vi "Keysight66332A.vi"(4 "error in":T13, 7 "Command":T14) -> (0 "error out":T13, 3 "Response":T11)   [LabVIEW 2018]
uses:
  MOKO_LabViewLibrary/MokoLowLevel/MokoLowLovelControl/MLLC_Command.ctl
  MOKO_LabViewLibrary/MokoLowLevel/MokoLowLovelControl/MLLC_Error.ctl
  MOKO_LabViewLibrary/MokoLowLevel/MokoLowLovelControl/MLLC_Mode.ctl
  MOKO_LabViewLibrary/MokoLowLevel/MokoLowLovelControl/MLLC_Response.ctl
  MOKO_LabViewLibrary/MokoLowLevel/MokoLowLovelControl/MLLC_DriverName.ctl
  MOKO_LabViewLibrary/MokoLowLevel/MokoLowLovelControl/MLLC_Request.ctl
  MOKO_LabViewLibrary/MokoLowLevel/MokoLowLovelControl/MLLC_ErrorCode.ctl
  MOKO_LabViewLibrary/MokoLowLevel/MokoLowLovelControl/MLLC_ResponseInit.ctl
  MOKO_LabViewLibrary/MokoLowLevel/MokoLowLovelControl/MLLC_ConnectCluster.ctl
  MOKO_LabViewLibrary/MokoLowLevel/MokoLowLovelControl/MLLC_InterfaceType.ctl
  MOKO_LabViewLibrary/MokoLowLevel/MokoLowLovelControl/MLLC_OpenedSession.ctl
  MOKO_LabViewLibrary/MokoLowLevel/MokoLowLovelControl/MLLC_InterfaceSettings.ctl
  MOKO_LabViewLibrary/MokoLowLevel/MokoLowLovelControl/MLLC_InterfaceKind.ctl
panel:
  in  "Settings":T6={"Saved Data"=variant, "Data"={"Connect"={"InterfaceType"=enum."VISA", "OpenedSession"="", "InterfaceSettings"={"Interface"=enum."GPIB", "EOS 4 read"=enum."LF (\\n)", "EOS 4 write"=enum."LF (\\n)", "TMO, ms"=5000, "Sett"=variant(cluster{"Baud Rate":u32, "Data Bits":u16, "Parity":u16, "Stop Bits":u16, "Flow Control":u16, "Eho":bool} {"Baud Rate"=75, "Data Bits"=0, "Parity"=0, "Stop Bits"=0, "Flow Control"=0, "Eho"=FALSE})}}, "VDC Range"=FALSE}}
  in  "Response":T7="663"
  in  "Error Code":T8=5475
  in  "Request":T9="*idn?"
  in  "Driver Name":T10="Keysight6632B"
  in  "Mode":T12=enum."Check"
  # ":VOLT:RANG LOW"
  # ":VOLT 5.000"
  # "SCPI = *RST"
  # "Keysight66332A"
  # "SCPI =OUTPut OFF"
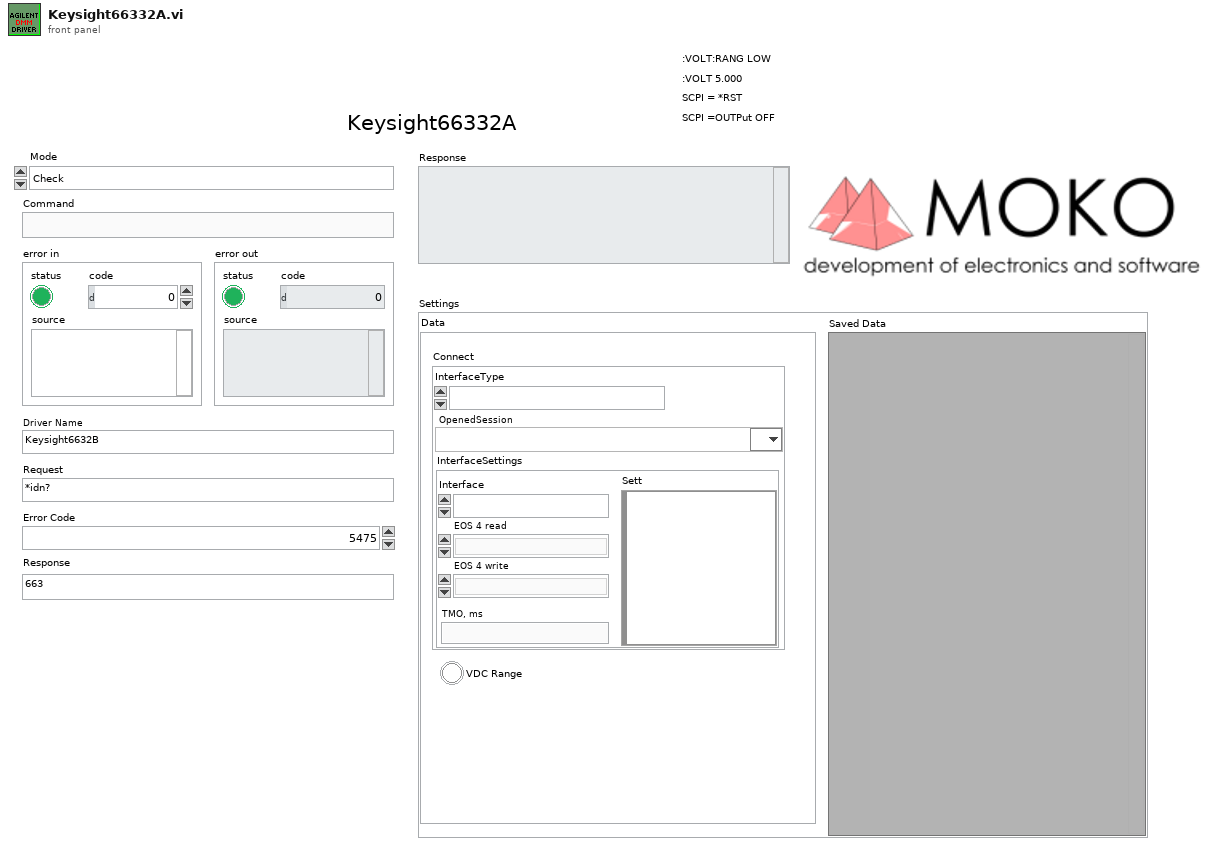
[diagram p1: front panel]
types:
  T1 = typedef "MLLC_ConnectCluster.ctl" = cluster{"InterfaceType":T2, "OpenedSession":T3, "InterfaceSettings":T4}
  T2 = typedef "MLLC_InterfaceType.ctl" = enum16{"VISA", "Prologix USB-GPIB"}
  T3 = typedef "MLLC_OpenedSession.ctl" = refnum<visa-resource-name>
  T4 = typedef "MLLC_InterfaceSettings.ctl" = cluster{"Interface":T5, "EOS 4 read":enum16{"Default (=EOS 4 write)", "CR (\\r)", "LF (\\n)", "None"}, "EOS 4 write":enum16{"CR+LF (\\r\\n)", "CR (\\r)", "LF (\\n)", "None"}, "TMO, ms":i32, "Sett":variant}
  T5 = typedef "MLLC_InterfaceKind.ctl" = enum16{"RS232", "GPIB", "USB", "Ethernet", "another"}
  T6 = cluster{"Saved Data":variant, "Data":cluster{"Connect":T1, "VDC Range":bool}}
  T7 = typedef "MLLC_ResponseInit.ctl" = string
  T8 = typedef "MLLC_ErrorCode.ctl" = u32
  T9 = typedef "MLLC_Request.ctl" = string
  T10 = typedef "MLLC_DriverName.ctl" = string
  T11 = typedef "MLLC_Response.ctl" = string
  T12 = typedef "MLLC_Mode.ctl" = enum16{"get", "set", "close", "Init", "Check"}
  T13 = typedef "MLLC_Error.ctl" = errorcluster
  T14 = typedef "MLLC_Command.ctl" = string
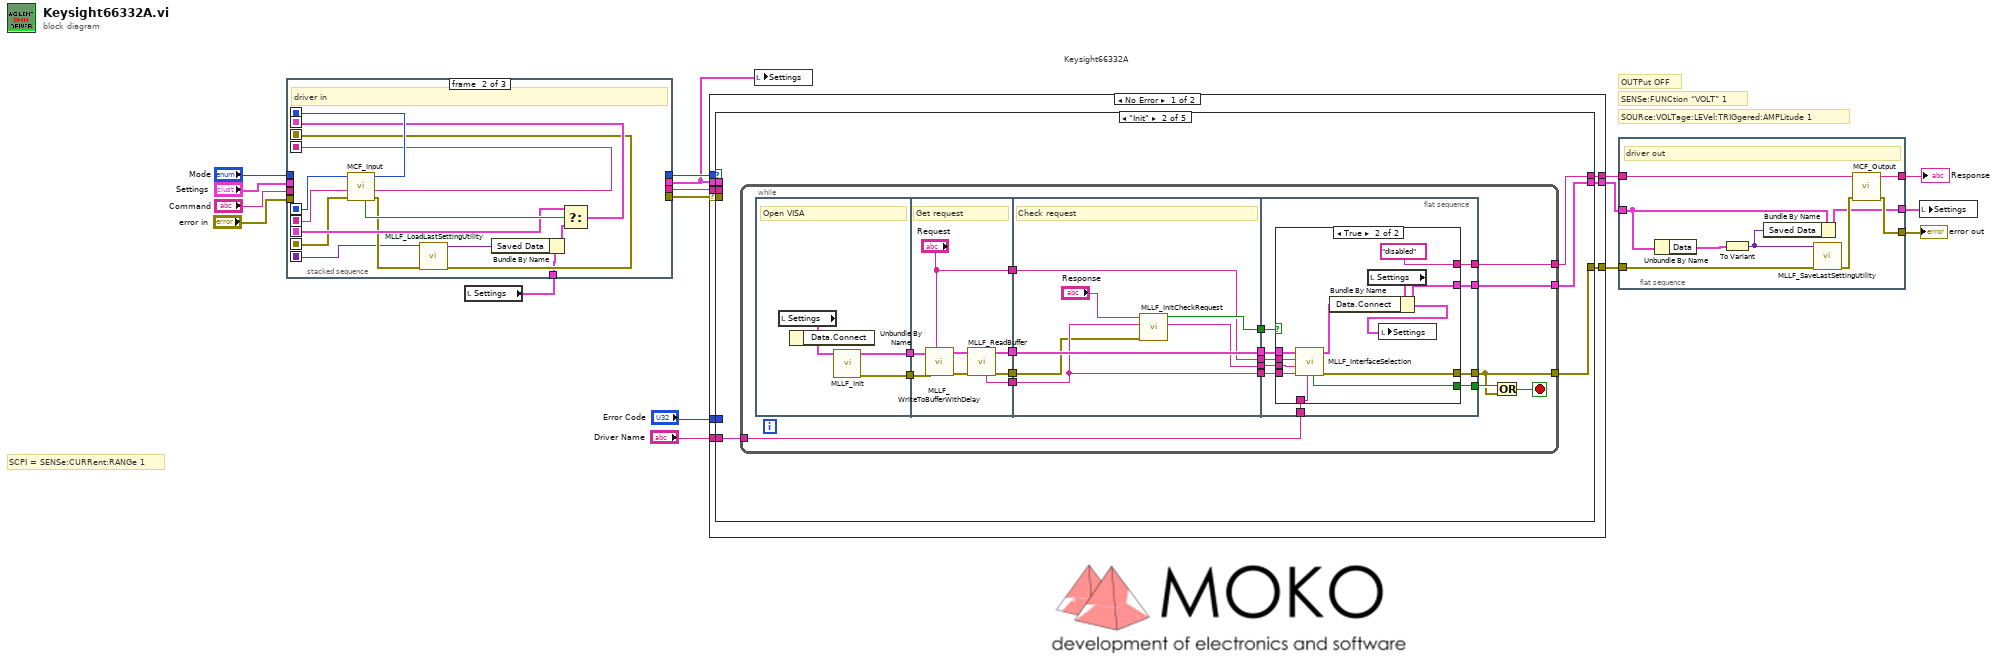
[diagram p0: block diagram]
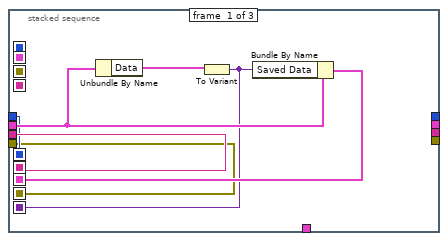
[diagram p2: hidden frame]
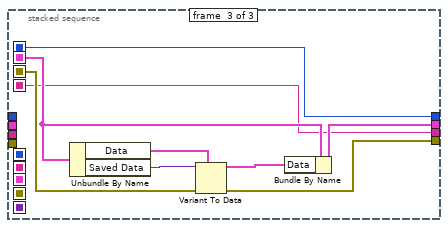
[diagram p3: hidden frame]
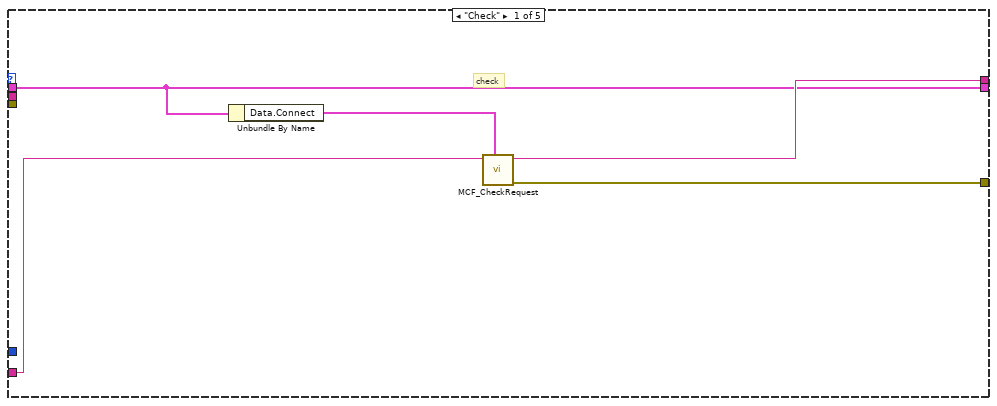
[diagram p4: hidden frame]
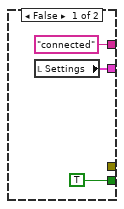
[diagram p5: hidden frame]
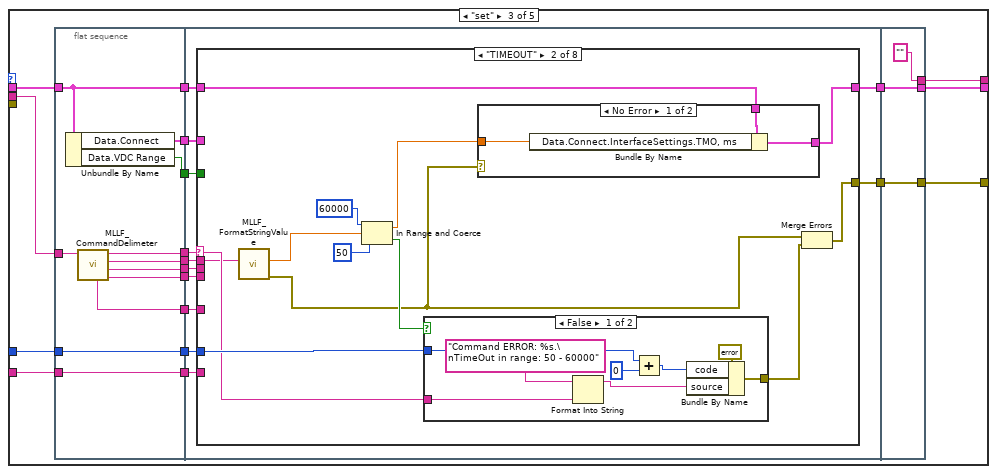
[diagram p6: hidden frame]
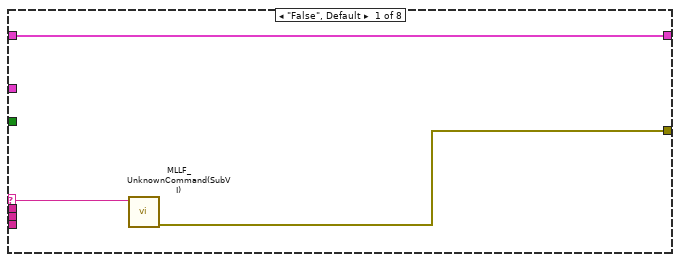
[diagram p7: hidden frame]
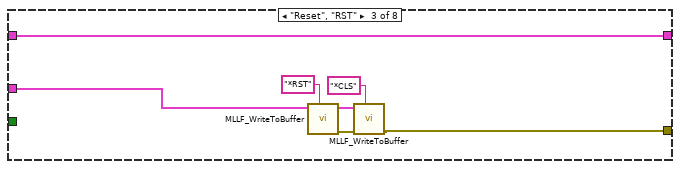
[diagram p10: hidden frame]
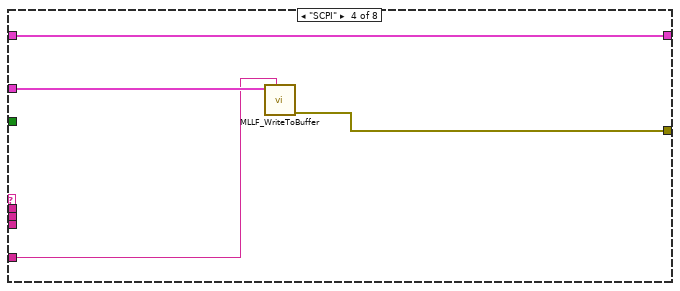
[diagram p11: hidden frame]
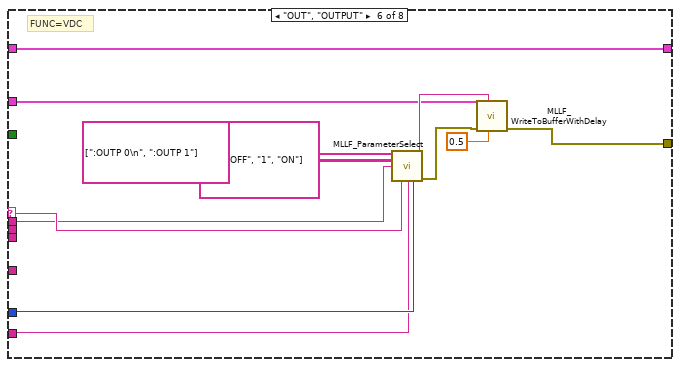
[diagram p13: hidden frame]
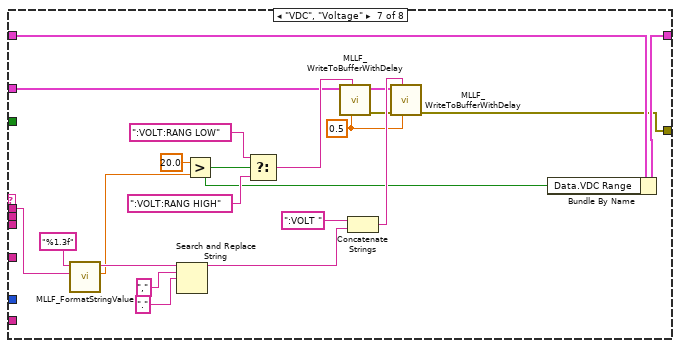
[diagram p14: hidden frame]
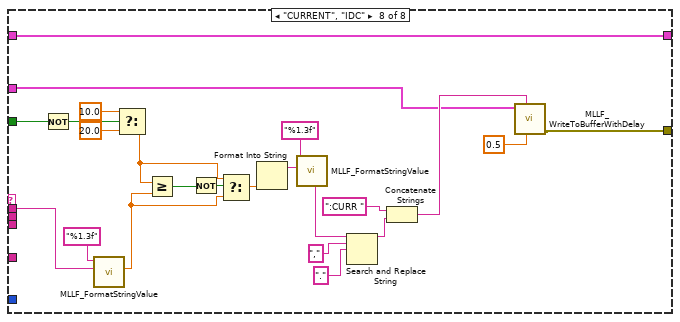
[diagram p15: hidden frame]
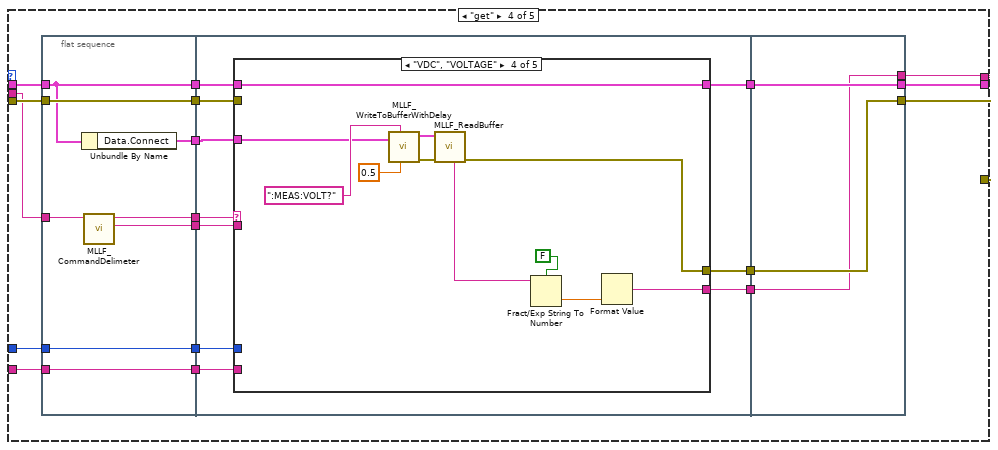
[diagram p16: hidden frame]
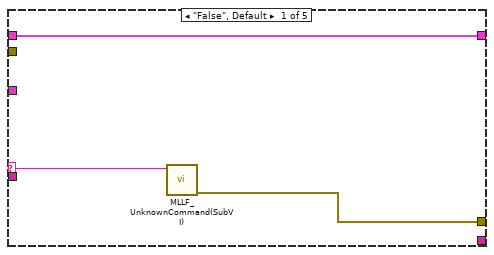
[diagram p17: hidden frame]
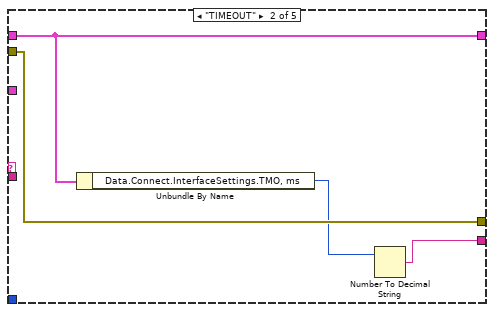
[diagram p18: hidden frame]
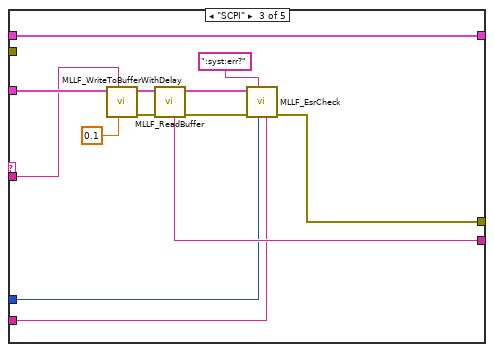
[diagram p19: hidden frame]
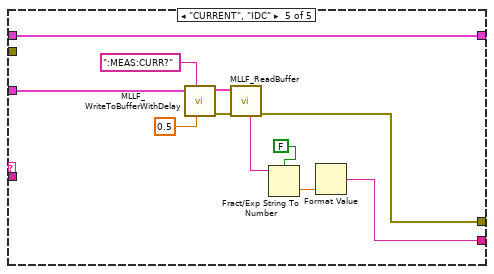
[diagram p20: hidden frame]
diagram:
  # "OUTPut OFF"
  # "SOURce:VOLTage:LEVel:TRIGgered:AMPLitude 1"
  # "SENSe:FUNCtion “VOLT” 1"
  # "SCPI = SENSe:CURRent:RANGe 1"
  # "Keysight66332A"
  n1 = local read "Settings"() -> (w8:T6)
  n2 = stacked-sequence {
    seq-local: [w20 _ _] -> [_ w36 _]
    seq-local: [w19 _ _] -> [_ w37 _]
    seq-local: [w22 _ _] -> [_ w32 _]
    seq-local: [w18 _ _] -> [_ w31 _]
    seq-local: [w21 _ _] -> [_ w27 _]
    seq-local: [_ w28 _] -> [_ _ w44]
    seq-local: [_ w38 _] -> [_ _ w41]
    seq-local: [_ w35 _] -> [_ _ w40]
    seq-local: [_ w34 _] -> [_ _ w45]
    tunnel: "Command" -> [w20 _ _]
    tunnel: "Mode" -> [w19 _ _]
    tunnel: "error in" -> [w18 _ _]
    tunnel: "Settings" -> [w23 _ _]
    tunnel: w8 -> [_ w26 _]
    tunnel: [_ _ w40] -> w10
    tunnel: [_ _ w43] -> w1
    tunnel: [_ _ w42] -> w9
    tunnel: [_ _ w41] -> w11
    frame #0 {
      n3 = Unbundle By Name(w23) -> ("Data"=w24:cluster{"Connect":T1, "VDC Range":bool})
      n4 = To Variant(anything=w24) -> (Variant=w21:variant)
      n5 = Bundle By Name(cluster=w23, "Saved Data"=w21) -> (w22:T6)
    }
    frame #1 {
      # "driver in"
      n6 = call "MCF_Input.vi"("Error In"=w31, "Command in"=w36, "Mode in"=w37) -> ("Error Out"=w30:errorcluster, "Command out"=w35:string, "Mode out"=w38:T12, "Boolean"=w33:bool)  [unwired: 5 in]
      n7 = call "MLLF_LoadLastSettingUtility.vi"("Error In"=w30, "Save data in"=w27) -> ("Error Out"=w28:errorcluster, "Save data out"=w25:variant)  [unwired: 8 in]
      n8 = Bundle By Name(cluster=w26, "Saved Data"=w25) -> (w29:T6)
      n9 = Select(t=w32, s=w33, f=w29) -> (s? t:f=w34:T6)
    }
    frame #2 {
      n10 = Unbundle By Name(w45) -> ("Data"=w46:cluster{"Connect":T1, "VDC Range":bool}, "Saved Data"=w39:variant)
      n11 = Variant To Data(error in=w44, type=w46, Variant=w39) -> (data=w47:cluster{"Connect":T1, "VDC Range":bool}, error out=w42:errorcluster)
      n12 = Bundle By Name(cluster=w45, "Data"=w47) -> (w43:T6)
    }
  }
  n13 = case shown="No Error" w9 {
    selector: w9 -> [w53 w354]
    tunnel: [w54 w354] -> w5
    tunnel: w11 -> [w56 _]
    tunnel: [w55 "An error occurred in the driver input module." ("String")] -> w7
    tunnel: w10 -> [w48 _]
    tunnel: w1 -> [w49 w353]
    tunnel: "Error Code" -> [w52 _]
    tunnel: "Driver Name" -> [w51 _]
    tunnel: [w50 w353] -> w6
    frame No Error {
      n14 = case shown="\"Init\"" w56 {
        tunnel: [w60 w65 w138 w267 "" ("String")] -> w55
        tunnel: [w61 w63 w141 w268 w350] -> w54
        tunnel: w53 -> [_ _ _ w281 _]
        tunnel: w52 -> [_ _ w144 w283 _]
        tunnel: w51 -> [w59 w62 w142 w282 _]
        tunnel: [w57 w64 w143 w284 w349] -> w50
        tunnel: w49 -> [w57 _ w129 w273 w349]
        tunnel: w48 -> [_ _ w128 w272 _]
        frame "Check" {
          # "check"
          n15 = Unbundle By Name(w57) -> ("Data.Connect"=w58:T1)
          n16 = call "MCF_CheckRequest.vi"("Permanent data.Connect"=w58, "Driver Name"=w59) -> ("Error Out"=w61:errorcluster, "Output String"=w60:string)  [unwired: 8 in]
        }
        frame "Init" {
          n17 = while {
            tunnel: [w71] -> w63
            tunnel: [w70] -> w65
            tunnel: [w69] -> w64
            tunnel: w62 -> [w73]
            stop <- w82 stop-if-true
            n18 = flat-sequence {
              tunnel: [w86] -> w81
              tunnel: [w85] -> w80
              tunnel: w81 -> [w92]
              tunnel: w80 -> [w91]
              tunnel: [w90] -> w79
              tunnel: [w89] -> w78
              tunnel: [w88] -> w77
              tunnel: ["Request"] -> w67
              tunnel: w79 -> [w98]
              tunnel: w78 -> [w101]
              tunnel: w77 -> [w100]
              tunnel: [w101] -> w76
              tunnel: [w100] -> w75
              tunnel: [w97] -> w74
              tunnel: [w96] -> w68
              tunnel: w67 -> [w95]
              tunnel: [w95] -> w66
              tunnel: w76 -> [w110]
              tunnel: w75 -> [w109]
              tunnel: w74 -> [w111]
              tunnel: w73 -> [w108]
              tunnel: [w107] -> w72
              tunnel: [w106] -> w71
              tunnel: [w105] -> w70
              tunnel: [w104] -> w69
              tunnel: w68 -> [w103]
              tunnel: w66 -> [w102]
              frame #0 {
                # "Open VISA"
                n19 = local read "Settings"() -> (w84:T6)
                n20 = Unbundle By Name(w84) -> ("Data.Connect"=w83:T1)
                n21 = call "MLLF_Init.vi"("DriverConnect in"=w83) -> ("Error Out"=w86:errorcluster, "DriverConnect out"=w85:T1)  [unwired: 7 in]
              }
              frame #1 {
                # "Get request"
                n22 = call "MLLF_WriteToBufferWithDelay.vi"("Command"="Request", "Error In"=w92, "DriverConnect in"=w91) -> ("Error Out"=w93:errorcluster, "DriverConnect out"=w94:T1)  [unwired: 7 in]
                n23 = call "MLLF_ReadBuffer.vi"("Error In"=w93, "DriverConnect in"=w94) -> ("Error Out"=w90:errorcluster, "DriverConnect out"=w89:T1, "String"=w88:string)  [unwired: 6 in]
              }
              frame #2 {
                # "Check request"
                n24 = call "MLLF_InitCheckRequest.vi"("error in (no error)"=w98, "Answer"=w100, "Response Init"="Response") -> ("ResponseInit out"=w96:string, "Design"=w97:bool)  [unwired: 5 in, 2 out]
              }
              frame #3 {
                n25 = case shown="True" w111 {
                  tunnel: w110 -> [_ w124]
                  tunnel: [TRUE w119] -> w107
                  tunnel: [_ w122] -> w106
                  tunnel: ["connected" "disabled"] -> w105
                  tunnel: [w112 w120] -> w104
                  tunnel: w109 -> [_ w117]
                  tunnel: w108 -> [_ w118]
                  tunnel: w103 -> [_ w116]
                  tunnel: w102 -> [_ w115]
                  frame False {
                    n26 = local read "Settings"() -> (w112:T6)
                  }
                  frame True {
                    n27 = call "MLLF_InterfaceSelection.vi"("Driver Name"=w118, "Answer:"=w117, "Response"=w116, "Request"=w115, "DriverConnect in"=w124) -> ("error out"=w122:T13, "DriverConnect out"=w123:T1, "stop init?"=w119:bool)  [unwired: 2 in, 2 out]
                    n28 = local read "Settings"() -> (w125:T6)
                    n29 = Bundle By Name(cluster=w125, "Data.Connect"=w123) -> (w120:T6)
                    n30 = local write "Settings"(w120) -> ()
                  }
                }
              }
            }
            n31 = Or(x=w72, y=w71) -> (x .or. y?=w82:bool)
          }
        }
        frame "set" {
          n32 = flat-sequence {
            tunnel: w142 -> [w154]
            tunnel: w129 -> [w147]
            tunnel: w144 -> [w155]
            tunnel: [w155] -> w137
            tunnel: [w147] -> w136
            tunnel: [w154] -> w135
            tunnel: [w153] -> w134
            tunnel: [w148] -> w133
            tunnel: [w149] -> w132
            tunnel: [w150] -> w131
            tunnel: [w151] -> w130
            tunnel: w128 -> [w152]
            tunnel: [w146] -> w127
            tunnel: [w145] -> w126
            tunnel: [w165] -> w140
            tunnel: [w160] -> w139
            tunnel: w137 -> [w167]
            tunnel: w136 -> [w166]
            tunnel: w135 -> [w164]
            tunnel: w134 -> [w163]
            tunnel: w133 -> [w162]
            tunnel: w132 -> [w161]
            tunnel: w131 -> [w159]
            tunnel: w130 -> [w158]
            tunnel: w127 -> [w157]
            tunnel: w126 -> [w156]
            tunnel: [w265] -> w141
            tunnel: [w266] -> w143
            tunnel: w140 -> [w266]
            tunnel: w139 -> [w265]
            tunnel: ["" ("String")] -> w138
            frame #0 {
              n33 = Unbundle By Name(w147) -> ("Data.Connect"=w153:T1, "Data.VDC Range"=w145:bool)
              n34 = call "MLLF_CommandDelimeter.vi"("command with param"=w152) -> ("param 3"=w151:string, "param 2"=w150:string, "param 1"=w149:string, "command"=w148:string, "Spit delimetre"=w146:string)  [unwired: 6 in]
            }
            frame #1 {
              n35 = case shown="\"TIMEOUT\"" w162 {
                selector: w162 -> [w169 w172 _ _ _ w210 _ _]
                tunnel: w161 -> [_ w171 _ _ _ w209 w225 w242]
                tunnel: [w168 w177 w196 w203 _ w208 w220 w241] -> w160
                tunnel: w167 -> [_ w178 _ _ _ w212 _ _]
                tunnel: w166 -> [w170 w182 w202 w206 w207 w219 w223 w247]
                tunnel: [w170 w183 w202 w206 w207 w219 w222 w247] -> w165
                tunnel: w163 -> [_ _ w197 w205 _ w213 w224 w246]
                tunnel: w164 -> [_ _ _ _ _ w211 _ _]
                tunnel: w159 -> [_ _ _ _ _ _ _ _]
                tunnel: w158 -> [_ _ _ _ _ _ _ _]
                tunnel: w157 -> [_ _ _ w204 _ _ _ _]
                tunnel: w156 -> [_ _ _ _ _ _ _ w245]
                frame "False", Default {
                  n36 = call "MLLF_UnknownCommand(SubVI).vi"("Unknown command"=w169) -> ("error out"=w168:errorcluster)  [unwired: 10 in]
                }
                frame "TIMEOUT" {
                  n37 = call "MLLF_FormatStringValue.vi"("String Value"=w171) -> ("error out"=w173:T13, "number"=w174:dbl)  [unwired: 8 in, 1 out]
                  n38 = In Range and Coerce(upper limit=60000, x=w174, lower limit=50) -> (coerced(x)=w179:dbl, In Range?=w175:bool)
                  n39 = case shown="False" w175 {
                    tunnel: [w190 _] -> w176
                    tunnel: w178 -> [w189 _]
                    tunnel: w172 -> [w188 _]
                    frame False {
                      n40 = Format Into String(format string="Command ERROR: %s.\nTimeOut in range: 50 - 60000", w188) -> (resulting string=w192:string)  [unwired: 2 in, 1 out]
                      n41 = Add(x=w189, y=0) -> (x+y=w193:T8)
                      n42 = Bundle By Name(cluster=errorcluster {"status"=TRUE, "code"=0, "source"=""} ("error out"), "code"=w193, "source"=w192) -> (w190:errorcluster)
                    }
                    frame True {
                    }
                  }
                  n43 = case shown="No Error" w173 {
                    tunnel: [w186 w187] -> w183
                    tunnel: w182 -> [w185 w187]
                    tunnel: w179 -> [w184 _]
                    frame No Error {
                      n44 = Bundle By Name(cluster=w185, "Data.Connect.InterfaceSettings.TMO, ms"=w184) -> (w186:T6)
                    }
                    frame Error {
                    }
                  }
                  n45 = Merge Errors(w173, w176) -> (w177:errorcluster)
                }
                frame "Reset", "RST" {
                  n46 = call "MLLF_WriteToBuffer.vi"("String"="*RST", "DriverConnect in"=w197) -> ("error out"=w200:T13, "DriverConnect out"=w201:T1)  [unwired: 6 in]
                  n47 = call "MLLF_WriteToBuffer.vi"("String"="*CLS" ("write buffer"), "error in"=w200, "DriverConnect in"=w201) -> ("error out"=w196:T13)  [unwired: 5 in, 1 out]
                }
                frame "SCPI" {
                  n48 = call "MLLF_WriteToBuffer.vi"("String"=w204, "DriverConnect in"=w205) -> ("error out"=w203:T13)  [unwired: 6 in, 1 out]
                }
                frame "<----MAIN FUNCTIONS---->" {
                }
                frame "OUT", "OUTPUT" {
                  # "FUNC=VDC"
                  n49 = call "MLLF_ParameterSelect.vi"("Command to equipment"=string[] [":OUTP 0\n", ":OUTP 1"] ("Names"), "Names"=string[][] [["0", "OFF"], ["1", "ON"]], "Input"=w209, "Command"=w210, "Driver Name"=w211, "Error Code"=w212) -> ("Choice"=w216:string, "Error Out"=w215:errorcluster)  [unwired: 8 in]
                  n50 = call "MLLF_WriteToBufferWithDelay.vi"("Delay Time ( 0,05 s)"=0.5 ("Delay Time (s)"), "Command"=w216, "Error In"=w215, "DriverConnect in"=w213) -> ("Error Out"=w208:errorcluster)  [unwired: 6 in, 1 out]
                }
                frame "VDC", "Voltage" {
                  w227 = 0.5 ("Delay Time (s)")
                  n51 = call "MLLF_FormatStringValue.vi"("String Value"=w225, "Format"="%1.3f" ("format string")) -> ("number"=w233:dbl, "String Value Formated"=w237:T14)  [unwired: 7 in, 1 out]
                  n52 = Search and Replace String(input string=w237, search string=",", replace string="." ("replace string (\"\")")) -> (result string=w235:string)  [unwired: 5 in, 3 out]
                  n53 = Greater?(x=20.0, y=w233) -> (0:w226:bool)
                  n54 = Select(t=":VOLT:RANG LOW" ("write buffer (\"\")"), s=w226, f=":VOLT:RANG HIGH" ("write buffer (\"\")")) -> (s? t:f=w228:string)
                  n55 = call "MLLF_WriteToBufferWithDelay.vi"("Delay Time ( 0,05 s)"=w227, "Command"=w228, "DriverConnect in"=w224) -> ("Error Out"=w231:errorcluster, "DriverConnect out"=w232:T1)  [unwired: 7 in]
                  n56 = Concatenate Strings(":VOLT " ("format string"), w235) -> (w234:string)
                  n57 = call "MLLF_WriteToBufferWithDelay.vi"("Delay Time ( 0,05 s)"=w227, "Command"=w234, "Error In"=w231, "DriverConnect in"=w232) -> ("Error Out"=w220:errorcluster)  [unwired: 6 in, 1 out]
                  n58 = Bundle By Name(cluster=w223, "Data.VDC Range"=w226) -> (w222:T6)
                }
                frame "CURRENT", "IDC" {
                  n59 = Not(x=w245) -> (.not. x?=w248:bool)
                  n60 = call "MLLF_FormatStringValue.vi"("String Value"=w242, "Format"="%1.3f" ("format string")) -> ("number"=w256:dbl)  [unwired: 7 in, 2 out]
                  n61 = Select(t=10.0, s=w248, f=20.0) -> (s? t:f=w253:dbl)
                  n62 = Greater Or Equal?(x=w253, y=w256) -> (x >= y?=w255:bool)
                  n63 = Not(x=w255) -> (.not. x?=w254:bool)
                  n64 = Select(t=w253, s=w254, f=w256) -> (s? t:f=w251:dbl)
                  n65 = Format Into String(w251) -> (resulting string=w250:string)  [unwired: 3 in, 1 out]
                  n66 = call "MLLF_FormatStringValue.vi"("String Value"=w250, "Format"="%1.3f" ("format string")) -> ("String Value Formated"=w249:T14)  [unwired: 7 in, 2 out]
                  n67 = Search and Replace String(input string=w249, search string=",", replace string="." ("replace string (\"\")")) -> (result string=w258:string)  [unwired: 5 in, 3 out]
                  n68 = Concatenate Strings(":CURR " ("format string"), w258) -> (w257:string)
                  n69 = call "MLLF_WriteToBufferWithDelay.vi"("Delay Time ( 0,05 s)"=0.5 ("Delay Time (s)"), "Command"=w257, "DriverConnect in"=w246) -> ("Error Out"=w241:errorcluster)  [unwired: 7 in, 1 out]
                }
              }
            }
            frame #2 {
            }
          }
        }
        frame "get" {
          n70 = flat-sequence {
            tunnel: w281 -> [w290]
            tunnel: w282 -> [w291]
            tunnel: w283 -> [w292]
            tunnel: w273 -> [w285]
            tunnel: [w285] -> w280
            tunnel: [w292] -> w279
            tunnel: [w291] -> w278
            tunnel: [w289] -> w277
            tunnel: [w286] -> w276
            tunnel: [w287] -> w275
            tunnel: [w290] -> w274
            tunnel: w272 -> [w288]
            tunnel: w280 -> [w302]
            tunnel: w279 -> [w300]
            tunnel: w278 -> [w299]
            tunnel: w277 -> [w297]
            tunnel: w276 -> [w296]
            tunnel: w275 -> [w295]
            tunnel: w274 -> [w293]
            tunnel: [w301] -> w271
            tunnel: [w298] -> w270
            tunnel: [w294] -> w269
            tunnel: [w347] -> w284
            tunnel: w271 -> [w347]
            tunnel: w270 -> [w346]
            tunnel: w269 -> [w345]
            tunnel: [w346] -> w268
            tunnel: [w345] -> w267
            frame #0 {
              n71 = Unbundle By Name(w285) -> ("Data.Connect"=w289:T1)
              n72 = call "MLLF_CommandDelimeter.vi"("command with param"=w288) -> ("param 1"=w287:string, "command"=w286:string)  [unwired: 6 in, 3 out]
            }
            frame #1 {
              n73 = case shown="\"VDC\", \"VOLTAGE\"" w296 {
                selector: w296 -> [w304 _ _ _ _]
                tunnel: [w303 w308 w310 w325 w336] -> w298
                tunnel: w300 -> [_ _ w312 _ _]
                tunnel: [w305 w309 w322 w333 w344] -> w301
                tunnel: w302 -> [w305 w309 w322 w333 w344]
                tunnel: w297 -> [_ _ w321 w326 w338]
                tunnel: w299 -> [_ _ w311 _ _]
                tunnel: w295 -> [_ _ w318 _ _]
                tunnel: [_ w306 w317 w323 w334] -> w294
                tunnel: w293 -> [_ w308 _ _ _]
                frame "False", Default {
                  n74 = call "MLLF_UnknownCommand(SubVI).vi"("Unknown command"=w304) -> ("error out"=w303:errorcluster)  [unwired: 10 in]
                }
                frame "TIMEOUT" {
                  n75 = Unbundle By Name(w309) -> ("Data.Connect.InterfaceSettings.TMO, ms"=w307:i32)
                  n76 = Number To Decimal String(number=w307) -> (decimal integer string=w306:string)  [unwired: 1 in]
                }
                frame "SCPI" {
                  n77 = call "MLLF_WriteToBufferWithDelay.vi"("Delay Time ( 0,05 s)"=0.1 ("Delay Time (s)"), "Command"=w318, "DriverConnect in"=w321) -> ("Error Out"=w320:errorcluster, "DriverConnect out"=w319:T1)  [unwired: 7 in]
                  n78 = call "MLLF_ReadBuffer.vi"("Error In"=w320, "DriverConnect in"=w319) -> ("Error Out"=w313:errorcluster, "DriverConnect out"=w314:T1, "String"=w317:string)  [unwired: 6 in]
                  n79 = call "MLLF_EsrCheck.vi"("Name"=w311, "Error code"=w312, "Error Query"=":syst:err?", "error in"=w313, "DriverConnect in"=w314) -> ("error out"=w310:T13)  [unwired: 5 in, 1 out]
                }
                frame "VDC", "VOLTAGE" {
                  n80 = call "MLLF_WriteToBufferWithDelay.vi"("Delay Time ( 0,05 s)"=0.5 ("Delay Time (s)"), "Command"=":MEAS:VOLT?" ("format string"), "DriverConnect in"=w326) -> ("Error Out"=w330:errorcluster, "DriverConnect out"=w331:T1)  [unwired: 7 in]
                  n81 = call "MLLF_ReadBuffer.vi"("Error In"=w330, "DriverConnect in"=w331) -> ("Error Out"=w325:errorcluster, "String"=w329:string)  [unwired: 6 in, 1 out]
                  n82 = Fract/Exp String To Number(use system decimal point (T)=FALSE, string=w329) -> (number=w324:dbl)  [unwired: 2 in, 1 out]
                  n83 = Format Value(value (0)=w324) -> (output string=w323:string)  [unwired: 2 in]
                }
                frame "CURRENT", "IDC" {
                  n84 = call "MLLF_WriteToBufferWithDelay.vi"("Delay Time ( 0,05 s)"=0.5 ("Delay Time (s)"), "Command"=":MEAS:CURR?" ("format string"), "DriverConnect in"=w338) -> ("Error Out"=w341:errorcluster, "DriverConnect out"=w342:T1)  [unwired: 7 in]
                  n85 = call "MLLF_ReadBuffer.vi"("Error In"=w341, "DriverConnect in"=w342) -> ("Error Out"=w336:errorcluster, "String"=w337:string)  [unwired: 6 in, 1 out]
                  n86 = Fract/Exp String To Number(use system decimal point (T)=FALSE, string=w337) -> (number=w335:dbl)  [unwired: 2 in, 1 out]
                  n87 = Format Value(value (0)=w335) -> (output string=w334:string)  [unwired: 2 in]
                }
              }
            }
            frame #2 {
            }
          }
        }
        frame "close" {
          n88 = Unbundle By Name(w349) -> ("Data.Connect.OpenedSession"=w351:T3)
          n89 = VISA Close(VISA resource name=w351) -> (error out=w350:errorcluster)  [unwired: 1 in]
        }
      }
    }
    frame Error {
    }
  }
  n90 = local write "Settings"(w1) -> ()
  n91 = flat-sequence {
    tunnel: [w363] -> w2
    tunnel: [w362] -> w4
    tunnel: w7 -> [w361]
    tunnel: w5 -> [w360]
    tunnel: w6 -> [w356]
    tunnel: [w358] -> w3
    frame #0 {
      # "driver out"
      n92 = Unbundle By Name(w356) -> ("Data"=w355:cluster{"Connect":T1, "VDC Range":bool})
      n93 = To Variant(anything=w355) -> (Variant=w357:variant)
      n94 = Bundle By Name(cluster=w356, "Saved Data"=w357) -> (w358:T6)
      n95 = call "MLLF_SaveLastSettingUtility.vi"("error in"=w360, "Saved Data"=w357) -> ("error out"=w359:T13)  [unwired: 8 in, 1 out]
      n96 = call "MCF_Output.vi"("Error In"=w359, "Input"=w361) -> ("Error Out"=w362:errorcluster, "Output"=w363:string)  [unwired: 8 in]
    }
  }
  n97 = local write "Settings"(w3) -> ()
  "error out" <- w4
  "Response" <- w2
